vi "Stop.vi"(8 "error in (no error)":errorcluster, 10 "Origin":string) -> (0 "error out":errorcluster)   [LabVIEW 2021, in "Temperature-Module.lvlib"]
doc: "Send the Stop request.\n_______\nCreated using Delacor User Event Scripter 1.0.0.6."
uses:
  Temperature-Module.lvlib
  Stop Argument--cluster.ctl
  <vilib>/event_ctls.llb/usereventprio.ctl
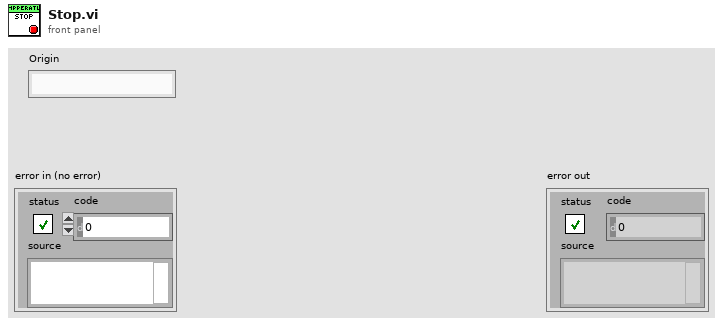
[diagram p1: front panel]
types:
  T1 = typedef "Temperature-Module.lvlib/Stop Argument--cluster.ctl" = cluster{"Origin":string}
  T2 = typedef "Temperature-Module.lvlib/Request Events--cluster.ctl" = cluster{"Stop":refnum<user-event>, "Start Temp Display":refnum<user-event>}
  T3 = typedef "usereventprio.ctl" = enum32{"high priority", "normal priority"}
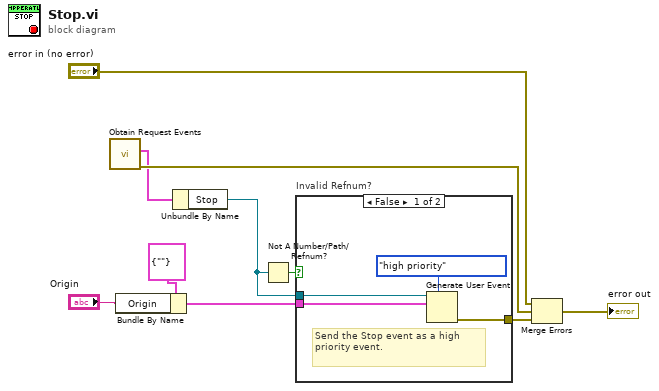
[diagram p0: block diagram]
diagram:
  n1 = call "Obtain Request Events.vi"() -> ("error out"=w7:errorcluster, "Temperature-Module Request Events"=w6:T2)  [unwired: 10 in]
  n2 = Bundle By Name(cluster=T1 {"Origin"=""} ("event data"), "Origin"="Origin") -> (w2:T1)
  n3 = Unbundle By Name(w6) -> ("Stop"=w3:refnum<user-event>)
  n4 = Not A Number/Path/Refnum?(number/path/refnum=w3) -> (NaN/Path/Refnum?=w4:bool)
  n5 = case "Invalid Refnum?" shown="False" w4 {
    tunnel: [w11 _] -> w1
    tunnel: w3 -> [w14 _]
    tunnel: w2 -> [w12 _]
    frame False {
      # "Send the Stop event as a high priority event."
      n6 = Generate User Event(priority (normal)=usereventprio."high priority", user event=w14, event data cluster=w12) -> (error out=w11:errorcluster)  [unwired: 1 in, 1 out]
    }
    frame True {
    }
  }
  n7 = Merge Errors("error in (no error)", w7, w1) -> (→"error out":errorcluster)
